vi "Construct Test Case.vi"(5 "Test Case in":refnum<class "Test Case.lvclass">, 8 "error in (no error)":errorcluster, 10 "Qualified Name":string, 11 "Path":path) -> (0 "error out":errorcluster, 3 "Test Case out":refnum<class "Test Case.lvclass">)   [LabVIEW 2017, in "Test Case.lvclass"]
uses:
  Test Case.lvclass
  Test Case.lvclass/Test Case.ctl
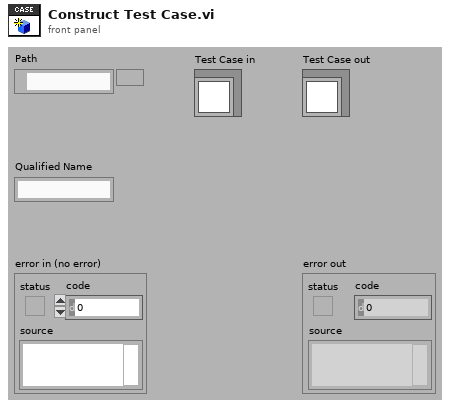
[diagram p1: front panel]
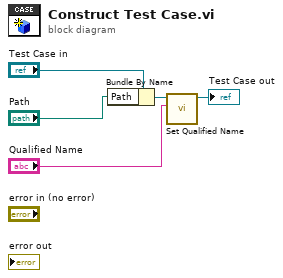
[diagram p0: block diagram]
diagram:
  n1 = Bundle By Name(cluster="Test Case in", "Path"="Path") -> (w4:refnum<class "Test Case.lvclass">)
  n2 = call "Set Qualified Name.vi"("Qualified Name"="Qualified Name", "Test Case in"=w4) -> ("Test Case out"=→"Test Case out":refnum<class "Test Case.lvclass">)  [unwired: 8 in, 1 out]
